vi "Delete_with_Check.vi"(1 "FilePath":path) -> (0 "Deleted Filepath":path)   [LabVIEW 2020]
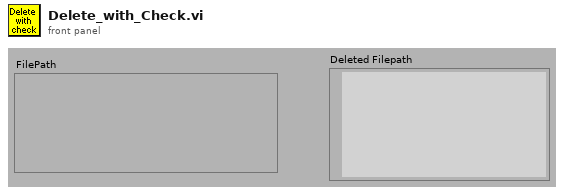
[diagram p1: front panel]
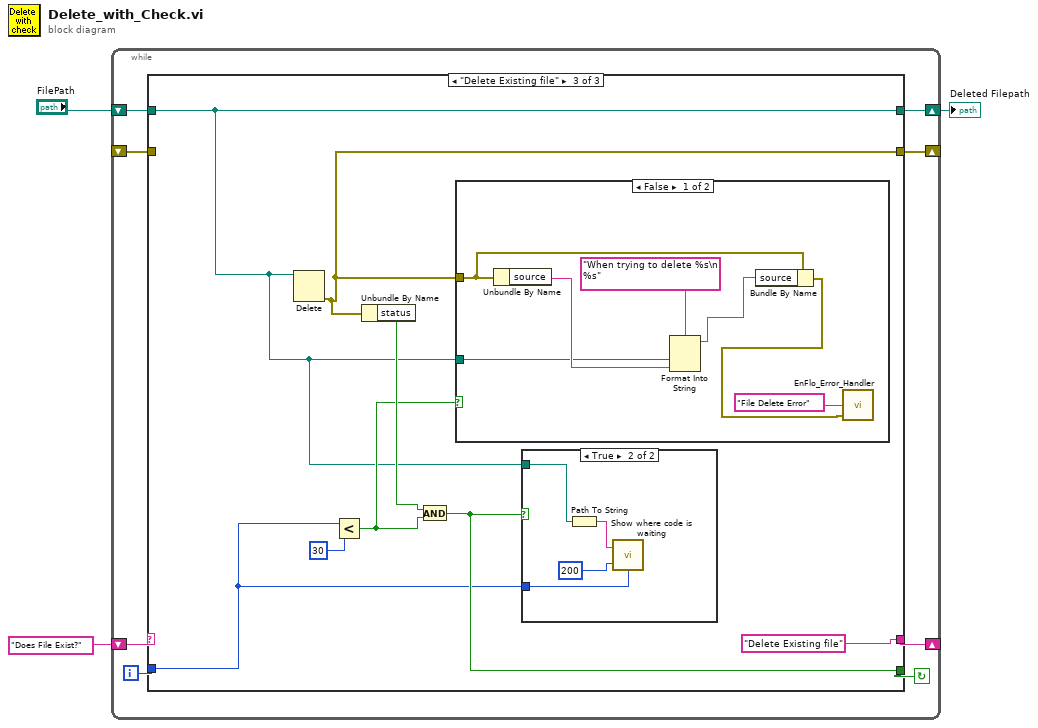
[diagram p0: block diagram]
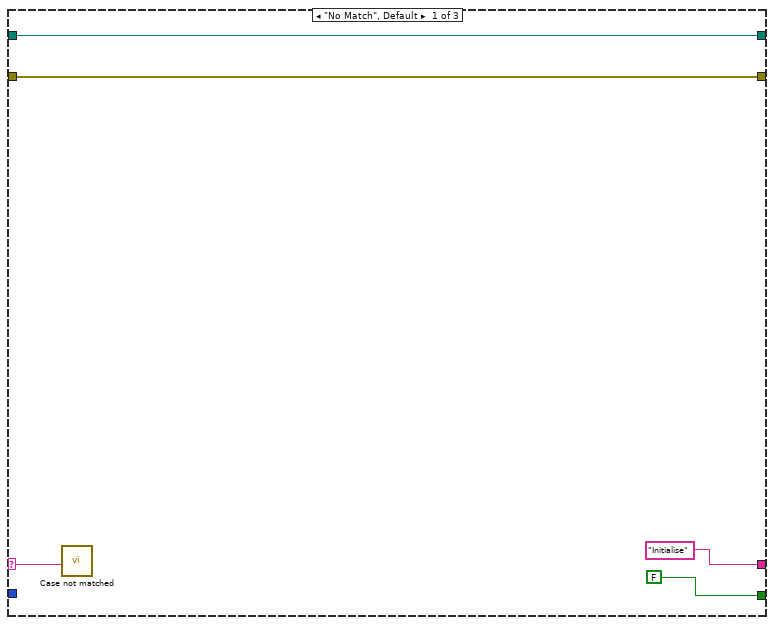
[diagram p2: hidden frame]
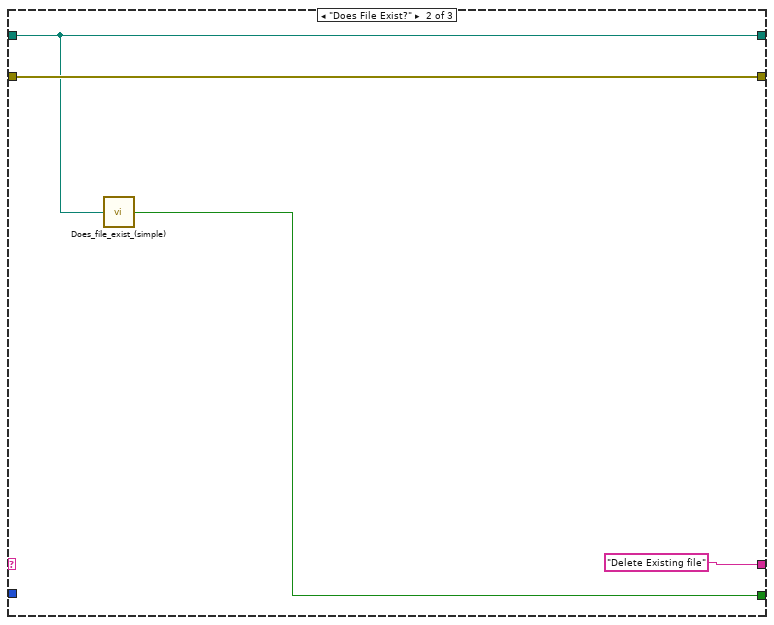
[diagram p3: hidden frame]
diagram:
  n1 = while {
    shift-left: "Does File Exist?" -> [w9]
    shift-right: [w10] -> _
    shift-right: [w7] -> w1
    shift-left: "FilePath" -> [w8]
    shift-right: [w6] -> _
    shift-left: _ -> [w5]
    i -> [w4]
    stop <- w11 continue-if-true
    n2 = case shown="\"Delete Existing file\"" w9 {
      selector: w9 -> [w12 _ _]
      tunnel: [FALSE w17 w23] -> w11
      tunnel: ["Initialise" "Delete Existing file" ("t") "Delete Existing file" ("t")] -> w10
      tunnel: w8 -> [w14 w19 w22]
      tunnel: [w14 w19 w22] -> w7
      tunnel: [w13 w20 w25] -> w6
      tunnel: w5 -> [w13 w20 _]
      tunnel: w4 -> [_ _ w21]
      frame "No Match", Default {
        n3 = call "Case not matched.vi"("Case Name not Matched"=w12) -> ()
      }
      frame "Does File Exist?" {
        n4 = call "Does_file_exist_(simple).vi"("Pathname"=w19) -> ("exists?"=w17:bool)
      }
      frame "Delete Existing file" {
        n5 = Delete(path (use dialog)=w22) -> (error out=w25:errorcluster)  [unwired: 1 in, 5 out]
        n6 = Less?(x=w21, y=30) -> (x < y?=w26:bool)
        n7 = Unbundle By Name(w25) -> ("status"=w27:bool)
        n8 = And(x=w27, y=w26) -> (x .and. y?=w23:bool)
        n9 = case shown="False" w26 {
          tunnel: w25 -> [w31 _]
          tunnel: w22 -> [w32 _]
          frame False {
            n10 = Unbundle By Name(w31) -> ("source"=w35:string)
            n11 = Format Into String(format string="When trying to delete %s\n %s", w32, w35) -> (resulting string=w33:string)  [unwired: 2 in, 1 out]
            n12 = Bundle By Name(cluster=w31, "source"=w33) -> (w29:errorcluster)
            n13 = call "EnFlo_Error_Handler.vi"("error in (no error)"=w29, "Error Type"="File Delete Error") -> ()  [unwired: 1 in, 3 out]
          }
          frame True {
          }
        }
        n14 = case shown="True" w23 {
          tunnel: w22 -> [_ w37]
          tunnel: w21 -> [_ w36]
          frame False {
          }
          frame True {
            n15 = Path To String(path=w37) -> (string=w39:string)
            n16 = call "Show where code is waiting.vi"("Loop index"=w36, "Wait (ms)"=u32 200 ("milliseconds to wait"), "Message"=w39) -> ()  [unwired: 1 in]
          }
        }
      }
    }
  }
  "Deleted Filepath" <- w1
